vi "Line sensor.vi"(8 "error in":errorcluster, 11 "FPGA VI Reference In":refnum<k20>) -> (0 "error out":errorcluster, 2 "appended array":bool[](array[boolean]), 3 "FPGA VI Reference Out":refnum<k20>)   [LabVIEW 2019]
uses:
  <vilib>/Utility/error.llb/Error Cluster From Error Code.vi
  <vilib>/rvi/errors/niLvFpgaAdjustHostInterfaceError.vi
  <vilib>/rvi/interface/nirviReadWriteControl/nirviReadWriteControl.xnode
  NiFpgaLv.dll
  <vilib>/rvi/interface/Simulation/niFpgaSimulationCallBeginRW.vi
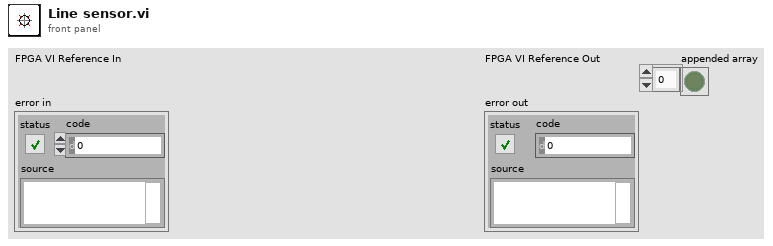
[diagram p1: front panel]
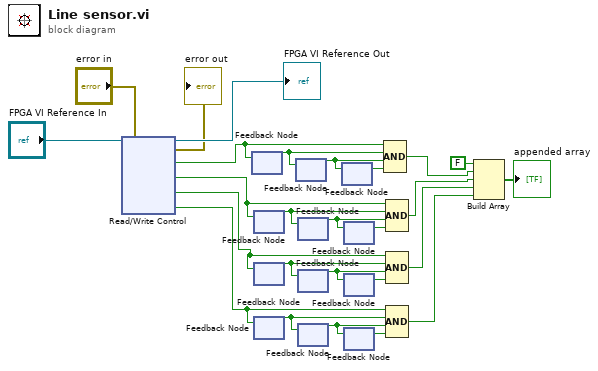
[diagram p0: block diagram]
diagram:
  n1 = xnode "Read/Write Control"("FPGA VI Reference In"="FPGA VI Reference In", "error in"="error in") -> ("FPGA VI Reference Out"=→"FPGA VI Reference Out":refnum<k20>, "error out"=→"error out":errorcluster, "Line 1"=w20:bool, "Line 2"=w12:bool, "Line 3"=w7:bool, "Line 4"=w1:bool)
  n2 = feedback-in #1(w20) -> ()
  n3 = feedback #1() -> (w19:bool)  [unwired: 1 in]
  n4 = feedback #2() -> (w13:bool)  [unwired: 1 in]
  n5 = feedback-in #2(w12) -> ()
  n6 = feedback #3() -> (w10:bool)  [unwired: 1 in]
  n7 = feedback-in #3(w7) -> ()
  n8 = feedback #4() -> (w3:bool)  [unwired: 1 in]
  n9 = feedback-in #4(w1) -> ()
  n10 = feedback #5() -> (w17:bool)  [unwired: 1 in]
  n11 = feedback-in #5(w19) -> ()
  n12 = feedback #6() -> (w14:bool)  [unwired: 1 in]
  n13 = feedback-in #6(w13) -> ()
  n14 = feedback #7() -> (w9:bool)  [unwired: 1 in]
  n15 = feedback-in #7(w10) -> ()
  n16 = feedback #8() -> (w4:bool)  [unwired: 1 in]
  n17 = feedback-in #8(w3) -> ()
  n18 = feedback #9() -> (w16:bool)  [unwired: 1 in]
  n19 = feedback-in #9(w17) -> ()
  n20 = feedback #10() -> (w15:bool)  [unwired: 1 in]
  n21 = feedback-in #10(w14) -> ()
  n22 = feedback #11() -> (w8:bool)  [unwired: 1 in]
  n23 = feedback-in #11(w9) -> ()
  n24 = feedback #12() -> (w5:bool)  [unwired: 1 in]
  n25 = feedback-in #12(w4) -> ()
  n26 = Compound Arithmetic op=AND(w20, w19, w17, w16) -> (w18:bool)
  n27 = Compound Arithmetic op=AND(w12, w13, w14, w15) -> (w11:bool)
  n28 = Compound Arithmetic op=AND(w7, w10, w9, w8) -> (w6:bool)
  n29 = Compound Arithmetic op=AND(w1, w3, w4, w5) -> (w2:bool)
  n30 = Build Array(FALSE ("element"), w18, w11, w6, w2) -> (→"appended array":bool[])
